vi "Set Port.vi"(8 "error in (no error)":errorcluster, 10 "Port":u16, 11 "URI in":refnum<class "URI.lvclass">) -> (0 "error out":errorcluster, 3 "URI out":refnum<class "URI.lvclass">)   [LabVIEW 2020, in "URI.lvclass"]
uses:
  URI.lvclass
  URI.lvclass/URI.ctl
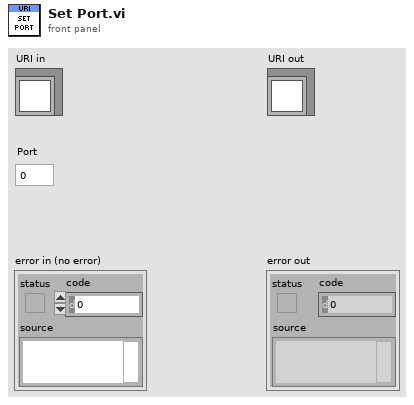
[diagram p1: front panel]
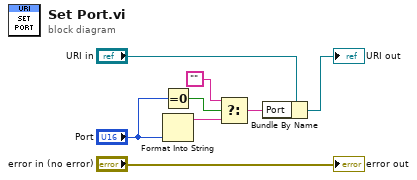
[diagram p0: block diagram]
diagram:
  n1 = Equal To 0?(x="Port") -> (x = 0?=w4:bool)
  n2 = Format Into String("Port") -> (resulting string=w3:string)  [unwired: 3 in, 1 out]
  n3 = Select(t="", s=w4, f=w3) -> (s? t:f=w1:string)
  n4 = Bundle By Name(cluster="URI in", "Port"=w1) -> (→"URI out":refnum<class "URI.lvclass">)
  "error out" <- "error in (no error)"
